vi "Write Responser.vi"(8 "error in (no error)":errorcluster, 9 "<JSON> response documentation":string, 10 "response cluster":variant, 11 "Help in":refnum<class "Help.lvclass">) -> (0 "error out":errorcluster, 3 "Help out":refnum<class "Help.lvclass">)   [LabVIEW 2019, in "Help.lvclass"]
uses:
  Help.lvclass
  Help.lvclass/Help.ctl
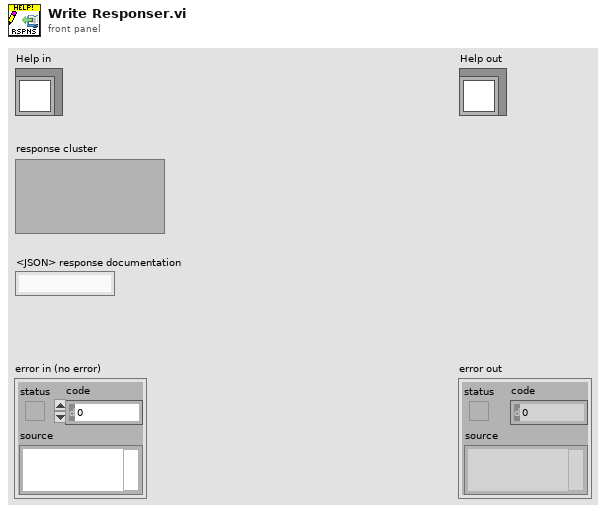
[diagram p1: front panel]
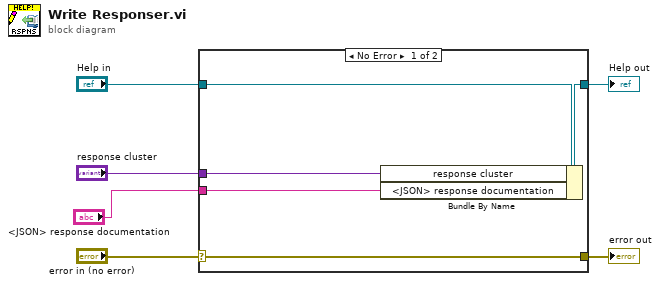
[diagram p0: block diagram]
diagram:
  n1 = case shown="No Error" "error in (no error)" {
    selector: "error in (no error)" -> [w11 w12]
    tunnel: [w11 w12] -> w5
    tunnel: [w9 w13] -> w3
    tunnel: "Help in" -> [w10 w13]
    tunnel: "response cluster" -> [w8 _]
    tunnel: "<JSON> response documentation" -> [w7 _]
    frame No Error {
      n2 = Bundle By Name(cluster=w10, "response cluster"=w8, "<JSON> response documentation"=w7) -> (w9:refnum<class "Help.lvclass">)
    }
    frame Error {
    }
  }
  "error out" <- w5
  "Help out" <- w3
